vi "SelectOne.vi"(8 "error in (no error)":errorcluster, 11 "ClassDataTree in":refnum<class "ClassDataTree.lvclass">) -> (0 "error out":errorcluster, 3 "ClassDataTree out":refnum<class "ClassDataTree.lvclass">)   [LabVIEW 2010, in "ClassDataTree.lvclass"]
uses:
  ClassDataTree.lvclass
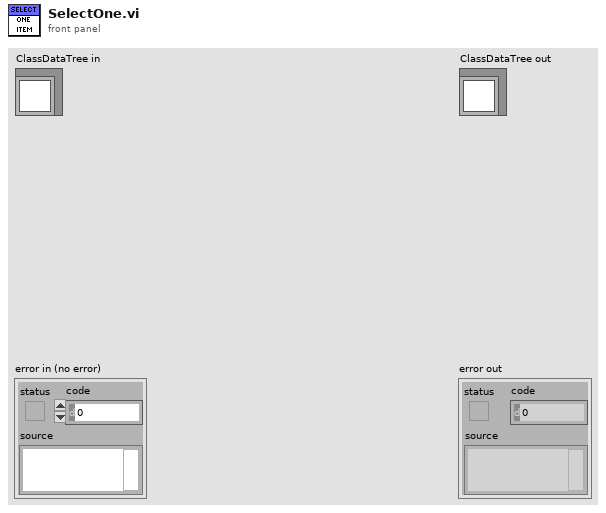
[diagram p1: front panel]
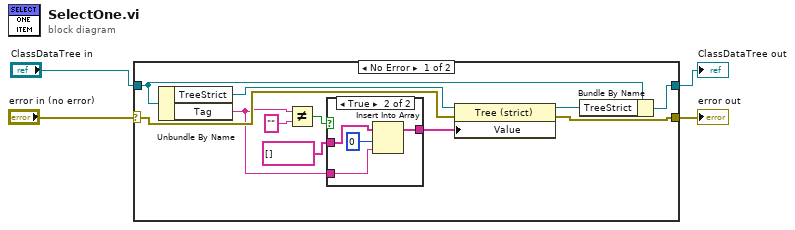
[diagram p0: block diagram]
diagram:
  n1 = case shown="No Error" "error in (no error)" {
    selector: "error in (no error)" -> [w14 w22]
    tunnel: [w13 w22] -> w3
    tunnel: [w10 w21] -> w1
    tunnel: "ClassDataTree in" -> [w12 w21]
    frame No Error {
      n2 = Unbundle By Name(w12) -> ("TreeStrict"=w15:refnum<vi>, "Tag"=w8:string)
      n3 = Not Equal?(x=w8, y="") -> (x != y?=w9:bool)
      n4 = case shown="True" w9 {
        tunnel: w8 -> [_ w20]
        tunnel: string[] [] ("Value") -> [w16 w18]
        tunnel: [w16 w17] -> w5
        frame False {
        }
        frame True {
          n5 = Insert Into Array(array=w18, index=0, new element=w20) -> (w17:string[])
        }
      }
      n6 = property class="Tree (strict)"(reference=w15, error in=w14, "Value"=w5) -> (reference out=w11:refnum<vi>, error out=w13:errorcluster)
      n7 = Bundle By Name(cluster=w12, "TreeStrict"=w11) -> (w10:refnum<class "ClassDataTree.lvclass">)
    }
    frame Error {
    }
  }
  "error out" <- w3
  "ClassDataTree out" <- w1
